vi "FPGA Get P2P FIFO Endpoint.vi"(8 "error in (no error)":errorcluster, 10 "FIFO":T1, 11 "FPGA Session In":refnum<class "Firmware Independent PID Interface.lvclass">) -> (0 "error out":errorcluster, 1 "Endpoint":u32, 3 "FPGA Session Out":refnum<class "Firmware Independent PID Interface.lvclass">)   [LabVIEW 2010, in "Firmware Independent PID Interface.lvclass"]
doc: "Gets an endpoint reference to a peer-to-peer FIFO."
uses:
  Firmware Independent PID Interface.lvclass
  TypeDefs/AllFifos.ctl
  <userlib>/_FPGA Interface Advanced Tools/FPGA Interface Base/FPGA Interface Base.lvclass/FPGA Interface Base.ctl
  <vilib>/Utility/error.llb/Error Cluster From Error Code.vi
  <userlib>/_FPGA Interface Advanced Tools/FPGA Interface Base/Accessors/FPGA Read Session.vi
  <userlib>/_FPGA Interface Advanced Tools/FPGA Interface Wrapper/FPGA Interface Wrapper.lvlib
  <userlib>/_FPGA Interface Advanced Tools/FPGA Interface Base/FPGA Interface Base.lvclass
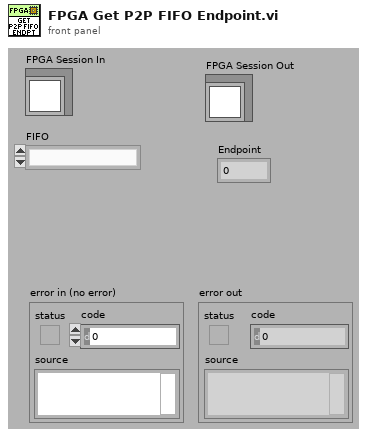
[diagram p1: front panel]
types:
  T1 = typedef "Firmware Independent PID Interface.lvclass/AllFifos.ctl" = enum16{""}
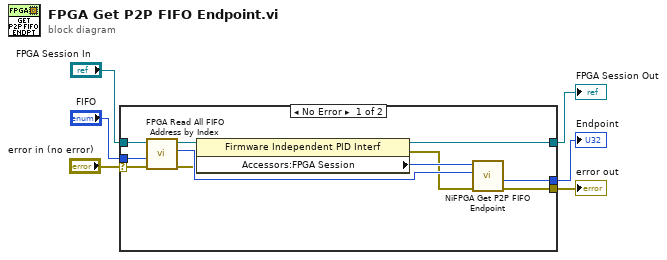
[diagram p0: block diagram]
diagram:
  n1 = case shown="No Error" "error in (no error)" {
    selector: "error in (no error)" -> [w16 w19]
    tunnel: [w9 w19] -> w1
    tunnel: [w10 w18] -> w3
    tunnel: "FPGA Session In" -> [w17 w18]
    tunnel: "FIFO" -> [w8 _]
    tunnel: [w7 _] -> w2
    frame No Error {
      n2 = call <userlib>:"FPGA Read All FIFO Address by Index.vi"("error in (no error)"=w16, "index"=w8, "FPGA Interface Base in"=w17) -> ("error out"=w13:errorcluster, "Address"=w15:u32, "FPGA Interface Base out"=w14:refnum<class "Firmware Independent PID Interface.lvclass">)  [unwired: 5 in, 1 out]
      n3 = property class="Firmware Independent PID Interf"(reference=w14, error in=w13) -> (reference out=w10:refnum<class "Firmware Independent PID Interface.lvclass">, error out=w11:errorcluster, "Accessors:FPGA Session"=w12:u32)
      n4 = call <userlib>:"NiFPGA Get P2P FIFO Endpoint.vi"("error in (no error)"=w11, "FIFO"=w15, "Session"=w12) -> ("error out"=w9:errorcluster, "Endpoint"=w7:u32)  [unwired: 6 in, 1 out]
    }
    frame Error {
    }
  }
  "error out" <- w1
  "FPGA Session Out" <- w3
  "Endpoint" <- w2
